vi "Read String Port COM.vi"(8 "entrée d'erreur":errorcluster={"status"=FALSE, "code"=0, "source"="L'opération s'est déroulée avec succès."} caption="entrée d'erreur (pas d'erreur)", 11 "Port d'entrée":refnum<visa-resource-name>="COM5") -> (0 "Sortie d'erreur":errorcluster={"status"=FALSE, "code"=1073676294, "source"="VISA Read dans ALR3220_GTBF.lvlib:Read_RS_R3220.vi->ALR3220_GTBF.lvlib:Wr_Rd_R3220.vi"} caption="sortie d'erreur", 2 "Réponse":string="0 OK\r", 3 "Port de sortie":refnum<visa-resource-name>="COM5", 5 "octets lus":u32=5)   [LabVIEW 2018]
doc: "Lecture sur le port série du nombre réel d'octets présents; grâce au caractère de terminaison (C.R, soit 0xD, soit \\r). \nPar la propriété “User Data”, qui a été chargée dans <B> 3206T_Init_RS.vi </B>\navec la taille du buffer d'entrée."
panel:
  # "© 2008 2018 elc  ALL RIGHTS RESERVED."
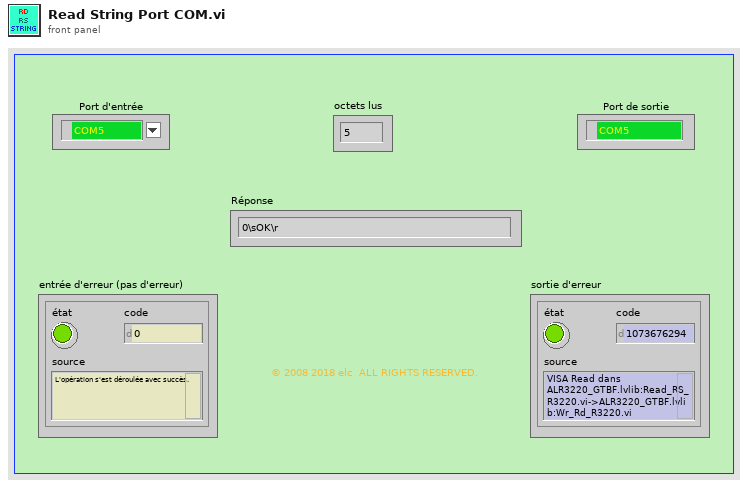
[diagram p1: front panel]
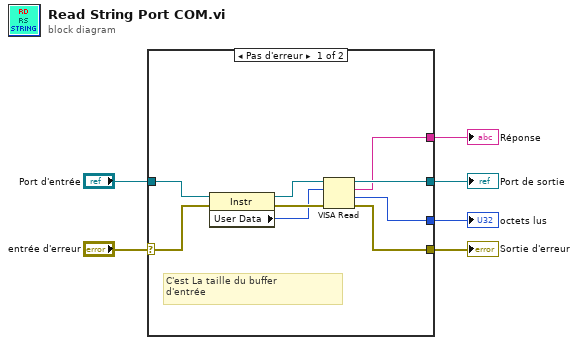
[diagram p0: block diagram]
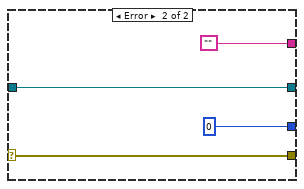
[diagram p2: hidden frame]
diagram:
  n1 = case shown="Pas d'erreur" "entrée d'erreur" {
    selector: "entrée d'erreur" -> [w12 w19]
    tunnel: [w14 w19] -> w6
    tunnel: [w15 w18] -> w5
    tunnel: "Port d'entrée" -> [w7 w18]
    tunnel: [w13 u32 0 ("return count")] -> w4
    tunnel: [w8 ""] -> w3
    frame No Error {
      # "C'est La taille du buffer\nd'entrée"
      n2 = property class="Instr"(reference=w7, error in=w12) -> (reference out=w11:refnum<visa-resource-name>, error out=w10:errorcluster, "User Data"=w9:u32)
      n3 = VISA Read(VISA resource name=w11, byte count=w9, error in (no error)=w10) -> (VISA resource name out=w15:refnum<visa-resource-name>, read buffer=w8:string, return count=w13:u32, error out=w14:errorcluster)
    }
    frame Error {
    }
  }
  "Sortie d'erreur" <- w6
  "Port de sortie" <- w5
  "Réponse" <- w3
  "octets lus" <- w4
